vi "Write Log Scan Progress.vi"(8 "error in (no error)":errorcluster, 10 "Scan Progress":T1 {"ILC Rate" format="%.3f"; "F Moment" format="%.3f"; "E Moment" format="%.3f"; "D Moment" format="%.3f"; "C Force" format="%.3f"; "B Force" format="%.3f"; "A Force" format="%.3f"; "Lateral Force" format="%.3f"; "Axial Force" format="%.3f"; "FC2 Measured Force" format="%.3f"; "FC1 Measured Force" format="%.3f"; "FC2 Demand" format="%.3f"; "FC1 Demand" format="%.3f"; "Lateral Demand" format="%.3f"; "Axial Demand" format="%.3f"}, 11 "Model in":refnum<class "Model.lvclass">) -> (0 "error out":errorcluster, 3 "Model out":refnum<class "Model.lvclass">)   [LabVIEW 2015, in "Model.lvclass"]
uses:
  Model.lvclass
  Typedefs/Scan Progress.ctl
  Typedefs/Cylinder Results.ctl
  Typedefs/Actuator Types.ctl
  Model.lvclass/Model.ctl
  Test Log/Test Log/Test Log.lvclass
  Typedefs/FAMT Typedefs.lvlib
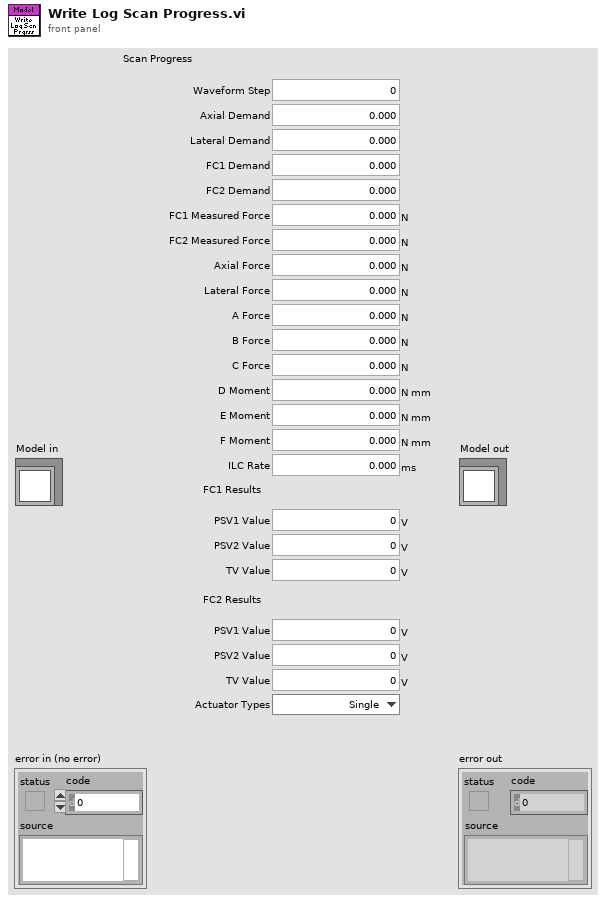
[diagram p1: front panel]
types:
  T1 = typedef "FAMT Typedefs.lvlib/Scan Progress.ctl" = cluster{"Waveform Step":u16, "Axial Demand":dbl, "Lateral Demand":dbl, "FC1 Demand":dbl, "FC2 Demand":dbl, "FC1 Measured Force":dbl[unit], "FC2 Measured Force":dbl[unit], "Axial Force":dbl[unit], "Lateral Force":dbl[unit], "A Force":dbl[unit], "B Force":dbl[unit], "C Force":dbl[unit], "D Moment":dbl[unit], "E Moment":dbl[unit], "F Moment":dbl[unit], "ILC Rate":dbl[unit], "FC1 Results":T2, "FC2 Results":T2, "Actuator Types":T3}
  T2 = typedef "FAMT Typedefs.lvlib/Cylinder Results.ctl" = cluster{"PSV1 Value":dbl[unit], "PSV2 Value":dbl[unit], "TV Value":dbl[unit]}
  T3 = typedef "FAMT Typedefs.lvlib/Actuator Types.ctl" = enum16{"Single", "Dual"}
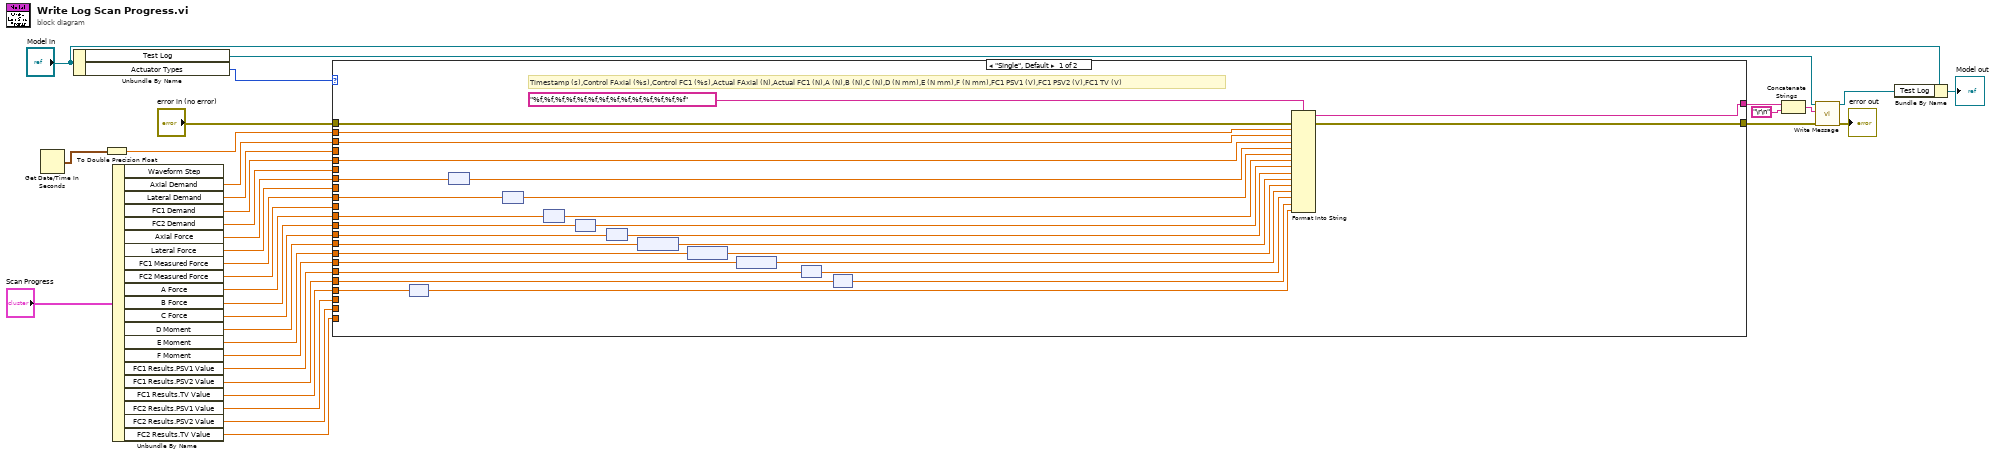
[diagram p0: block diagram]
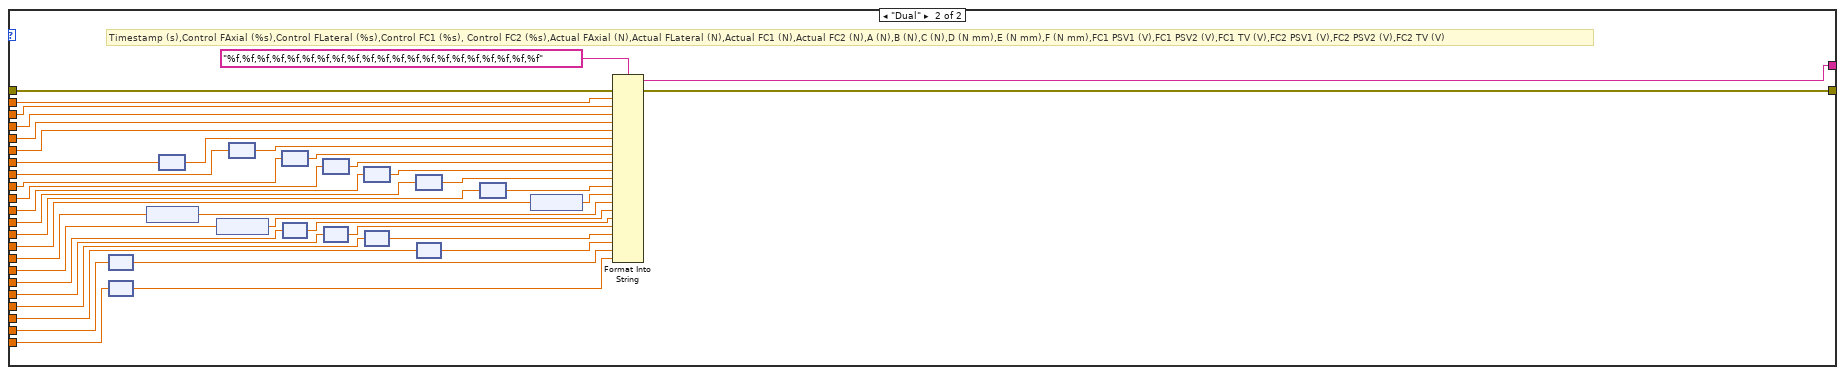
[diagram p2: hidden frame]
diagram:
  n1 = Get Date/Time In Seconds() -> (seconds since 1Jan1904=w26:timestamp)
  n2 = Unbundle By Name("Model in") -> ("Test Log"=w27:refnum<class "Test Log.lvclass">, "Actuator Types"=w32:T3)
  n3 = To Double Precision Float(number=w26) -> (double precision float=w25:dbl)
  n4 = Unbundle By Name("Scan Progress") -> ("Axial Demand"=w23:dbl, "Lateral Demand"=w22:dbl, "FC1 Demand"=w21:dbl, "FC2 Demand"=w20:dbl, "Axial Force"=w19:dbl[unit], "Lateral Force"=w18:dbl[unit], "FC1 Measured Force"=w17:dbl[unit], "FC2 Measured Force"=w16:dbl[unit], "A Force"=w15:dbl[unit], "B Force"=w14:dbl[unit], "C Force"=w13:dbl[unit], "D Moment"=w12:dbl[unit], "E Moment"=w11:dbl[unit], "F Moment"=w10:dbl[unit], "FC1 Results.PSV1 Value"=w6:dbl[unit], "FC1 Results.PSV2 Value"=w5:dbl[unit], "FC1 Results.TV Value"=w4:dbl[unit], "FC2 Results.PSV1 Value"=w3:dbl[unit], "FC2 Results.PSV2 Value"=w2:dbl[unit], "FC2 Results.TV Value"=w1:dbl[unit])  [unwired: 1 out]
  n5 = case shown="\"Single\", Default" w32 {
    tunnel: [w60 w101] -> w8
    tunnel: "error in (no error)" -> [w61 w103]
    tunnel: [w62 w102] -> w29
    tunnel: w25 -> [w59 w90]
    tunnel: w23 -> [w50 w89]
    tunnel: w22 -> [_ w88]
    tunnel: w21 -> [w49 w87]
    tunnel: w20 -> [_ w86]
    tunnel: w19 -> [w51 w93]
    tunnel: w18 -> [_ w92]
    tunnel: w17 -> [w52 w94]
    tunnel: w16 -> [_ w91]
    tunnel: w15 -> [w53 w95]
    tunnel: w14 -> [w54 w96]
    tunnel: w13 -> [w55 w97]
    tunnel: w12 -> [w56 w98]
    tunnel: w11 -> [w57 w99]
    tunnel: w10 -> [w58 w100]
    tunnel: w6 -> [w40 w71]
    tunnel: w5 -> [w39 w72]
    tunnel: w4 -> [w38 w73]
    tunnel: w3 -> [_ w74]
    tunnel: w2 -> [_ w75]
    tunnel: w1 -> [_ w76]
    frame "Single", Default {
      # "Timestamp (s),Control FAxial (%s),Control FC1 (%s),Actual FAxial (N),Actual FC1 (N),A (N),B (N),C (N),D (N mm),E (N mm),F (N mm),FC1 PSV1 (V),FC1 PSV2 (V),FC1 TV (V)"
      n6 = node(w38) -> (w37:dbl)
      n7 = node(w51) -> (w48:dbl)
      n8 = node(w52) -> (w47:dbl)
      n9 = node(w53) -> (w46:dbl)
      n10 = node(w54) -> (w45:dbl)
      n11 = node(w55) -> (w44:dbl)
      n12 = node(w56) -> (w43:dbl)
      n13 = node(w57) -> (w42:dbl)
      n14 = node(w58) -> (w41:dbl)
      n15 = node(w40) -> (w35:dbl)
      n16 = node(w39) -> (w36:dbl)
      n17 = Format Into String(format string="%f,%f,%f,%f,%f,%f,%f,%f,%f,%f,%f,%f,%f,%f", error in=w61, w59, w50, w49, w48, w47, w46, w45, w44, w43, w42, w41, w35, w36, w37) -> (resulting string=w60:string, error out=w62:errorcluster)  [unwired: 1 in]
    }
    frame "Dual" {
      # "Timestamp (s),Control FAxial (%s),Control FLateral (%s),Control FC1 (%s), Control FC2 (%s),Actual FAxial (N),Actual FLateral (N),Actual FC1 (N),Actual FC2 (N),A (N),B (N),C (N),D (N mm),E (N mm),F (N mm),FC1 PSV1 (V),FC1 PSV2 (V),FC1 TV (V),FC2 PSV1 (V),FC2 PSV2 (V),FC2 TV (V)"
      n18 = node(w75) -> (w65:dbl)
      n19 = node(w76) -> (w64:dbl)
      n20 = node(w99) -> (w77:dbl)
      n21 = node(w93) -> (w85:dbl)
      n22 = node(w100) -> (w70:dbl)
      n23 = node(w92) -> (w84:dbl)
      n24 = node(w94) -> (w83:dbl)
      n25 = node(w71) -> (w69:dbl)
      n26 = node(w91) -> (w82:dbl)
      n27 = node(w72) -> (w68:dbl)
      n28 = node(w95) -> (w81:dbl)
      n29 = node(w73) -> (w67:dbl)
      n30 = node(w96) -> (w80:dbl)
      n31 = node(w74) -> (w66:dbl)
      n32 = node(w97) -> (w79:dbl)
      n33 = node(w98) -> (w78:dbl)
      n34 = Format Into String(format string="%f,%f,%f,%f,%f,%f,%f,%f,%f,%f,%f,%f,%f,%f,%f,%f,%f,%f,%f,%f,%f", error in=w103, w90, w89, w88, w87, w86, w85, w84, w83, w82, w81, w80, w79, w78, w77, w70, w69, w68, w67, w66, w65, w64) -> (resulting string=w101:string, error out=w102:errorcluster)  [unwired: 1 in]
    }
  }
  n35 = Concatenate Strings(w8, "\r\n") -> (w7:string)
  n36 = call-dynamic "Write Message.vi"("error in (no error)"=w29, "Message"=w7, "Test Log in"=w27) -> ("error out"=→"error out":errorcluster, "Test Log out"=w30:refnum<class "Test Log.lvclass">)  [unwired: 7 in]
  n37 = Bundle By Name(cluster="Model in", "Test Log"=w30) -> (→"Model out":refnum<class "Model.lvclass">)
